vi "Get DMA FIFO to Target Name.vi"(5 "Expected Image Type":T1 items=["Grayscale (U8)", "Grayscale (I16)", "Grayscale (SGL)", "Complex (CSG)", "RGB (U32)", "HSL (U32)", "RGB (U64)", "Grayscale (U16)"], 6 "DMA FIFO Depth in Images":u32, 7 "Resource Names":T2, 8 "error in (no error)":errorcluster, 9 "Image Size":T3, 10 "Image":T4, 11 "FPGA Refnum In":refnum<k20>) -> (0 "error out":errorcluster, 1 "DMA FIFO Size":u32, 2 "DMA FIFO to Target Name":string, 3 "Refnum out":refnum<k20>)   [LabVIEW 2020, in "NI_VDM_FPGA_Basics.lvlib"]
uses:
  <vilib>/visionFPGA/NI_VDM_FPGA_Basics.lvlib
  <vilib>/vision/Image Controls.llb/IMAQ Image.ctl
  <vilib>/visionFPGA/Controls/IMAQ FPGA Image Size.ctl
  <vilib>/NI/LVFPGA Adv Session Resources/LVFPGAAdvSessionResources.lvlib
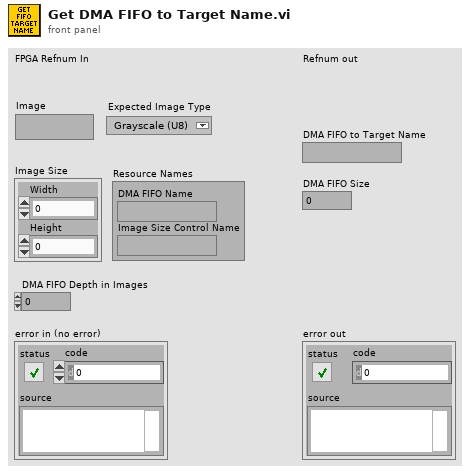
[diagram p1: front panel]
types:
  T1 = typedef "Image Type" = u32
  T2 = cluster{"DMA FIFO Name":string, "Image Size Control Name":string}
  T3 = typedef "IMAQ FPGA Image Size.ctl" = cluster{"Width":u32, "Height":u32}
  T4 = typedef "IMAQ Image.ctl" = refnum<image>
  T5 = enum16{"Register", "Host To Target FIFO", "Target To Host FIFO"}
  T6 = typedef "LVFPGAAdvSessionResources.lvlib/ResourceInfo.ctl" = cluster{"Resource name":string, "Data type":variant, "Resource type":enum16{"Register", "Host To Target FIFO", "Target To Host FIFO"}}
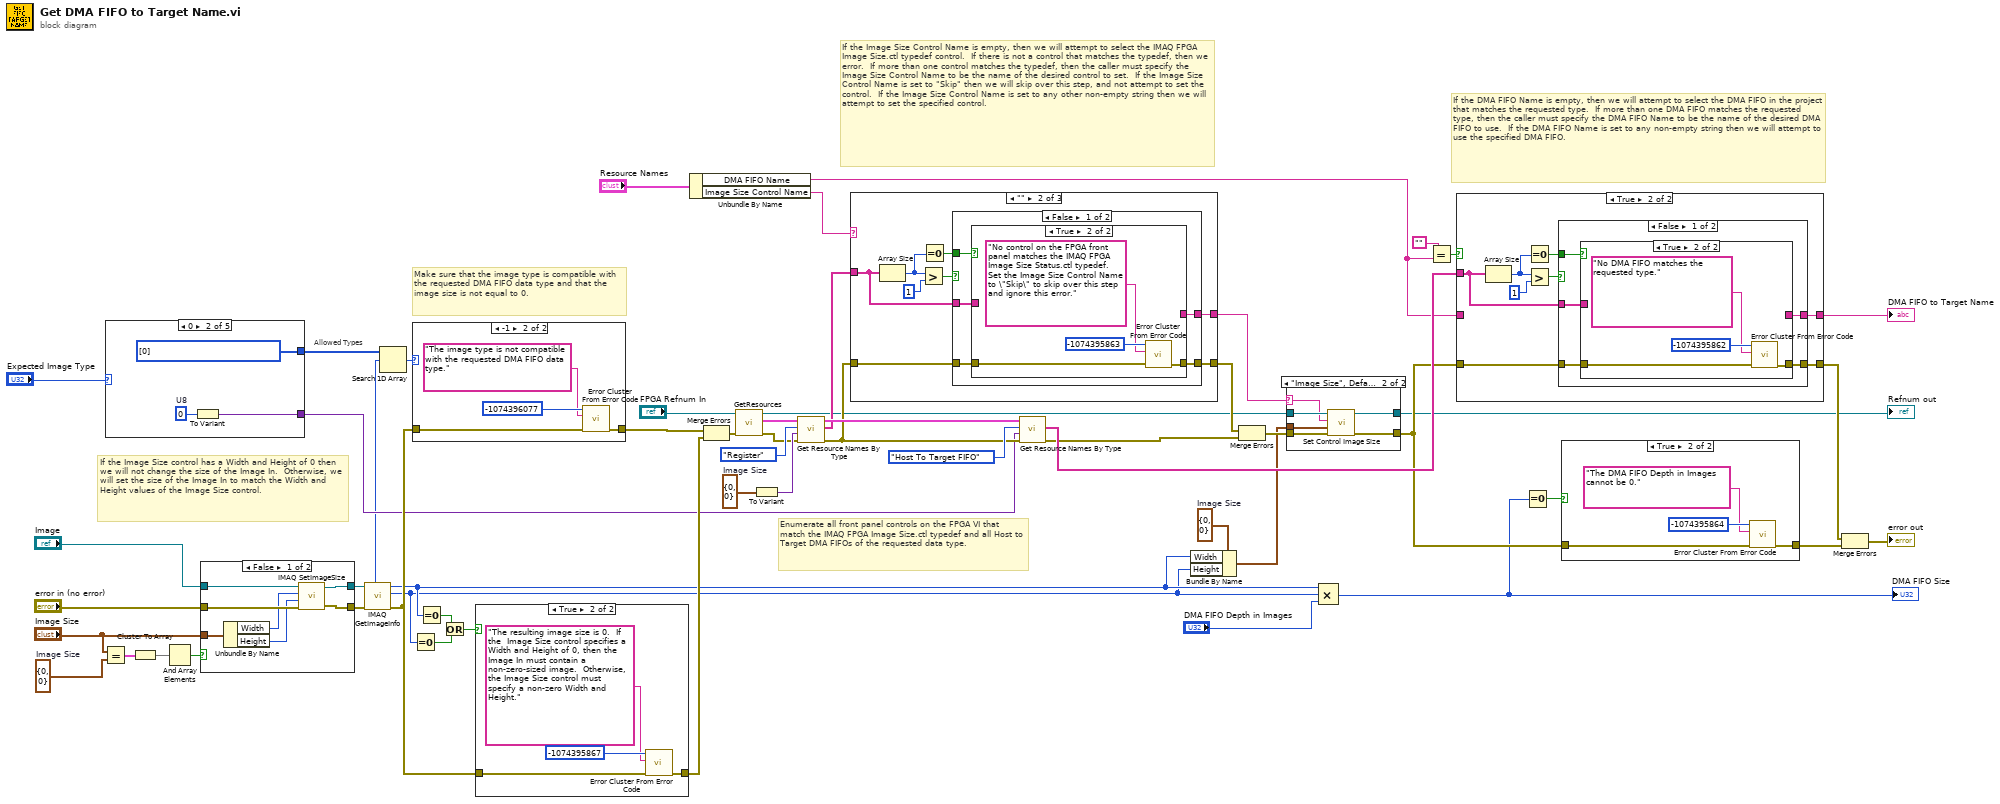
[diagram p0: block diagram]
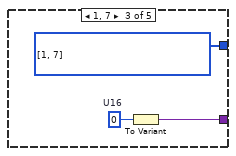
[diagram p3: hidden frame]
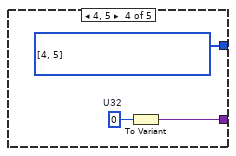
[diagram p4: hidden frame]
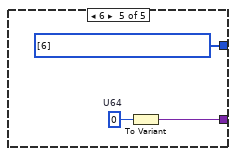
[diagram p5: hidden frame]
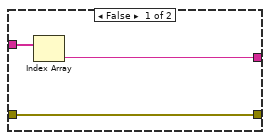
[diagram p11: hidden frame]
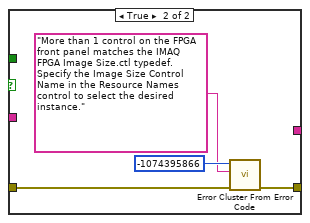
[diagram p12: hidden frame]
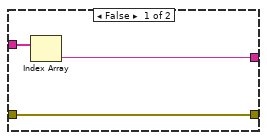
[diagram p15: hidden frame]
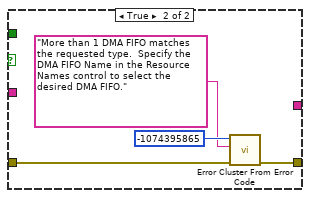
[diagram p16: hidden frame]
diagram:
  w24 = T3 {"Width"=0, "Height"=0}  # Image Size
  w19 = T3 {"Width"=0, "Height"=0}  # Image Size
  w18 = T3 {"Width"=0, "Height"=0}  # Image Size
  # "Allowed Types"
  # "Make sure that the image type is compatible with the requested DMA FIFO data type and that the image size is not equal to 0."
  # "If the Image Size control has a Width and Height of 0 then we will not change the size of the Image In.  Otherwise, we will set the size of the Image In to match the Width and Height values of the Image Size control."
  # "If the DMA FIFO Name is empty, then we will attempt to select the DMA FIFO in the project that matches the requested type.  If more than one DMA FIFO matches the requested type, then the caller must specify the DMA FIFO Name to be the name of the desired DMA FIFO to use.  If the DMA FIFO Name is set to any non-empty string then we will attempt to use the specified DMA FIFO."
  # "Enumerate all front panel controls on the FPGA VI that match the IMAQ FPGA Image Size.ctl typedef and all Host to Target DMA FIFOs of the requested data type."
  # "If the Image Size Control Name is empty, then we will attempt to select the IMAQ FPGA Image Size.ctl typedef control.  If there is not a control that matches the typedef, then we error.  If more than one control matches the typedef, then the caller must specify the Image Size Control Name to be the name of the desired control to set.  If the Image Size Control Name is set to \"Skip\" then we will skip over this step, and not attempt to set the control.  If the Image Size Control Name is set to any other non-empty string then we will attempt to set the specified control."
  n1 = Equal?(x="Image Size", y=w24) -> (x = y?=w21:cluster{"Width":bool, "Height":bool})
  n2 = case shown="0" "Expected Image Type" {
    tunnel: [_ w57 w59 w62 w65] -> w4
    tunnel: [_ w56 w61 w64 w67] -> w3
    frame Default {
      # "Undefined type. Pass empty array of valid types."
    }
    frame 0 {
      w56 = T1[] [0] items=["Grayscale (U8)", "Grayscale (I16)", "Grayscale (SGL)", "Complex (CSG)", "RGB (U32)", "HSL (U32)", "RGB (U64)", "Grayscale (U16)"]
      w58 = u8 0  # U8
      n3 = To Variant(anything=w58) -> (Variant=w57:variant)
    }
    frame 1, 7 {
      w60 = u16 0  # U16
      w61 = T1[] [1, 7] items=["Grayscale (U8)", "Grayscale (I16)", "Grayscale (SGL)", "Complex (CSG)", "RGB (U32)", "HSL (U32)", "RGB (U64)", "Grayscale (U16)"]
      n4 = To Variant(anything=w60) -> (Variant=w59:variant)
    }
    frame 4, 5 {
      w63 = u32 0  # U32
      w64 = T1[] [4, 5] items=["Grayscale (U8)", "Grayscale (I16)", "Grayscale (SGL)", "Complex (CSG)", "RGB (U32)", "HSL (U32)", "RGB (U64)", "Grayscale (U16)"]
      n5 = To Variant(anything=w63) -> (Variant=w62:variant)
    }
    frame 6 {
      w66 = u64 0  # U64
      w67 = T1[] [6] items=["Grayscale (U8)", "Grayscale (I16)", "Grayscale (SGL)", "Complex (CSG)", "RGB (U32)", "HSL (U32)", "RGB (U64)", "Grayscale (U16)"]
      n6 = To Variant(anything=w66) -> (Variant=w65:variant)
    }
  }
  n7 = Cluster To Array(cluster=w21) -> (array=w22:bool[])
  n8 = And Array Elements(Boolean array=w22) -> (logical AND=w23:bool)
  n9 = case shown="False" w23 {
    tunnel: "Image Size" -> [w72 _]
    tunnel: "Image" -> [w74 w76]
    tunnel: "error in (no error)" -> [w73 w75]
    tunnel: [w69 w76] -> w26
    tunnel: [w68 w75] -> w27
    frame False {
      n10 = Unbundle By Name(w72) -> ("Width"=w71:u32, "Height"=w70:u32)
      n11 = call "IMAQ SetImageSize"("error in (no error)"=w73, "Y Resolution"=w70, "X Resolution"=w71, "Image"=w74) -> ("error out"=w68:errorcluster, "Image Out"=w69:T4)  [unwired: 1 in]
    }
    frame True {
    }
  }
  n12 = call "IMAQ GetImageInfo"("error in (no error)"=w27, "Image"=w26) -> ("error out"=w35:errorcluster, "Y Resolution"=w30:i32, "X Resolution"=w31:i32, "Image Type"=w2:T1)  [unwired: 2 in, 4 out]
  n13 = Search 1D Array(1D array=w3, element=w2) -> (index of element=w1:i32)  [unwired: 1 in]
  n14 = Equal To 0?(x=w30) -> (x = 0?=w33:bool)
  n15 = case shown="-1" w1 {
    tunnel: w35 -> [w77 w79]
    tunnel: [w77 w78] -> w36
    frame Default {
    }
    frame -1 {
      n16 = call <vilib>:"Error Cluster From Error Code.vi"("error in (no error)"=w79, "error message (\"\")"="The image type is not compatible with the requested DMA FIFO data type." ("error message (\"\")"), "error code (0)"=-1074396077) -> ("error out"=w78:errorcluster)  [unwired: 6 in]
    }
  }
  n17 = Equal To 0?(x=w31) -> (x = 0?=w32:bool)
  n18 = Or(x=w32, y=w33) -> (x .or. y?=w34:bool)
  n19 = case shown="True" w34 {
    tunnel: w35 -> [w82 w84]
    tunnel: [w82 w83] -> w38
    frame False {
    }
    frame True {
      n20 = call <vilib>:"Error Cluster From Error Code.vi"("error in (no error)"=w84, "error message (\"\")"="The resulting image size is 0.  If the  Image Size control specifies a Width and Height of 0, then the Image In must contain a non-zero-sized image.  Otherwise, the Image Size control must specify a non-zero Width and Height." ("error message (\"\")"), "error code (0)"=-1074395867) -> ("error out"=w83:errorcluster)  [unwired: 6 in]
    }
  }
  n21 = Unbundle By Name("Resource Names") -> ("DMA FIFO Name"=w9:string, "Image Size Control Name"=w17:string)
  n22 = Merge Errors(w36, w38) -> (w37:errorcluster)
  n23 = call <vilib>:"GetResources.vi"("error in (no error)"=w37, "FPGA VI Reference in"="FPGA Refnum In") -> ("error out"=w20:errorcluster, "Resource info out"=w50:T6[], "FPGA VI Reference out"=w13:refnum<k20>)  [unwired: 7 in]
  n24 = To Variant(anything=w18) -> (Variant=w47:variant)
  n25 = call <vilib>:"Get Resource Names By Type.vi"("error in (no error)"=w20, "Data Type"=w47, "Resource Type"=T5."Register", "Resource Info In"=w50) -> ("error out"=w49:errorcluster, "Resource Names"=w53:string[], "Resource Info Out (dup)"=w54:T6[])  [unwired: 5 in]
  n26 = case shown="\"\"" w17 {
    selector: w17 -> [w87 _ _]
    tunnel: w49 -> [w88 w95 w113]
    tunnel: [w88 w94 w113] -> w39
    tunnel: [w87 w93 _] -> w15
    tunnel: w53 -> [_ w91 _]
    frame "Anything Else", Default {
    }
    frame "" {
      n27 = Array Size(array=w91) -> (size(s)=w90:i32)
      n28 = Greater?(x=w90, y=1 ("x")) -> (0:w96:bool)
      n29 = Equal To 0?(x=w90) -> (x = 0?=w89:bool)
      n30 = case shown="False" w96 {
        tunnel: w91 -> [w101 _]
        tunnel: [w100 _] -> w93
        tunnel: [w98 w110] -> w94
        tunnel: w95 -> [w99 w109]
        tunnel: w89 -> [w97 _]
        frame False {
          n31 = case shown="True" w97 {
            tunnel: w101 -> [w104 _]
            tunnel: [w103 _] -> w100
            tunnel: w99 -> [w102 w105]
            tunnel: [w102 w106] -> w98
            frame False {
              n32 = Index Array(array=w104) -> (element=w103:string)  [unwired: 1 in]
            }
            frame True {
              n33 = call <vilib>:"Error Cluster From Error Code.vi"("error in (no error)"=w105, "error message (\"\")"="No control on the FPGA front panel matches the IMAQ FPGA Image Size Status.ctl typedef.  Set the Image Size Control Name to \"Skip\" to skip over this step and ignore this error." ("error message (\"\")"), "error code (0)"=-1074395863) -> ("error out"=w106:errorcluster)  [unwired: 6 in]
            }
          }
        }
        frame True {
          n34 = call <vilib>:"Error Cluster From Error Code.vi"("error in (no error)"=w109, "error message (\"\")"="More than 1 control on the FPGA front panel matches the IMAQ FPGA Image Size.ctl typedef.  Specify the Image Size Control Name in the Resource Names control to select the desired instance." ("error message (\"\")"), "error code (0)"=-1074395866) -> ("error out"=w110:errorcluster)  [unwired: 6 in]
        }
      }
    }
    frame "Skip" {
    }
  }
  n35 = call <vilib>:"Get Resource Names By Type.vi"("error in (no error)"=w49, "Data Type"=w4, "Resource Type"=T5."Host To Target FIFO", "Resource Info In"=w54) -> ("error out"=w52:errorcluster, "Resource Names"=w55:string[])  [unwired: 5 in, 1 out]
  n36 = Bundle By Name(cluster=w19, "Width"=w31, "Height"=w30) -> (w14:T3)
  n37 = Merge Errors(w39, w52) -> (w40:errorcluster)
  n38 = case shown="\"Image Size\", Default" w15 {
    selector: w15 -> [_ w117]
    tunnel: [w115 w121] -> w16
    tunnel: [w114 w120] -> w43
    tunnel: w40 -> [w114 w119]
    tunnel: w13 -> [w115 w118]
    tunnel: w14 -> [_ w116]
    frame "" {
    }
    frame "Image Size", Default {
      n39 = call <vilib>:"Set Control Image Size.vi"("error in (no error)"=w119, "Image Size"=w116, "FPGA Control Name"=w117, "FPGA VI Reference In"=w118) -> ("error out"=w120:errorcluster, "FPGA VI Reference Out"=w121:refnum<k20>)  [unwired: 6 in]
    }
  }
  "Refnum out" <- w16
  n40 = Compound Arithmetic op=MULTIPLY(w31, w30, "DMA FIFO Depth in Images") -> (w42:u32)
  "DMA FIFO Size" <- w42
  n41 = Equal?(x="", y=w9) -> (x = y?=w8:bool)
  n42 = case shown="True" w8 {
    tunnel: w55 -> [_ w128]
    tunnel: w43 -> [w122 w127]
    tunnel: [w122 w130] -> w44
    tunnel: [w123 w129] -> w10
    tunnel: w9 -> [w123 _]
    frame False {
    }
    frame True {
      n43 = Array Size(array=w128) -> (size(s)=w124:i32)
      n44 = Greater?(x=w124, y=1 ("x")) -> (0:w126:bool)
      n45 = Equal To 0?(x=w124) -> (x = 0?=w125:bool)
      n46 = case shown="False" w126 {
        tunnel: w128 -> [w136 _]
        tunnel: [w135 _] -> w129
        tunnel: [w133 w145] -> w130
        tunnel: w127 -> [w134 w144]
        tunnel: w125 -> [w132 _]
        frame False {
          n47 = case shown="True" w132 {
            tunnel: w136 -> [w139 _]
            tunnel: [w138 _] -> w135
            tunnel: w134 -> [w137 w140]
            tunnel: [w137 w141] -> w133
            frame False {
              n48 = Index Array(array=w139) -> (element=w138:string)  [unwired: 1 in]
            }
            frame True {
              n49 = call <vilib>:"Error Cluster From Error Code.vi"("error in (no error)"=w140, "error message (\"\")"="No DMA FIFO matches the requested type." ("error message (\"\")"), "error code (0)"=-1074395862) -> ("error out"=w141:errorcluster)  [unwired: 6 in]
            }
          }
        }
        frame True {
          n50 = call <vilib>:"Error Cluster From Error Code.vi"("error in (no error)"=w144, "error message (\"\")"="More than 1 DMA FIFO matches the requested type.  Specify the DMA FIFO Name in the Resource Names control to select the desired DMA FIFO." ("error message (\"\")"), "error code (0)"=-1074395865) -> ("error out"=w145:errorcluster)  [unwired: 6 in]
        }
      }
    }
  }
  "DMA FIFO to Target Name" <- w10
  n51 = Equal To 0?(x=w42) -> (x = 0?=w41:bool)
  n52 = case shown="True" w41 {
    tunnel: [w148 w150] -> w45
    tunnel: w43 -> [w148 w149]
    frame False {
    }
    frame True {
      n53 = call <vilib>:"Error Cluster From Error Code.vi"("error in (no error)"=w149, "error message (\"\")"="The DMA FIFO Depth in Images cannot be 0." ("error message (\"\")"), "error code (0)"=-1074395864) -> ("error out"=w150:errorcluster)  [unwired: 6 in]
    }
  }
  n54 = Merge Errors(w44, w45) -> (→"error out":errorcluster)
